vi "ADC_spb.vi"(1 "18_1":i8=18, 2 "18_1":i8=18, 3 "8":i8=8, 4 "7":i8=7, 5 "Write Data":bool[](array[boolean])=[FALSE, FALSE, FALSE, FALSE, FALSE, FALSE, FALSE, FALSE, FALSE], 6 "Enum":T1(ring)=enum."GREEN OFF", 7 "Read(T)/Write(F)":bool, 8 "Command array":bool[](array[boolean])=[FALSE, FALSE, FALSE, FALSE, FALSE, FALSE, FALSE, FALSE, FALSE, FALSE, FALSE, FALSE, FALSE, FALSE, FALSE, FALSE, FALSE]) -> (0 "READ":bool[](array[boolean]))   [LabVIEW 2018]
uses:
  <vilib>/Platform/TimedLoop/XDataNode/timing_clust.ctl
  <vilib>/Platform/TimedLoop/XDataNode/nitl_modes.ctl
  <vilib>/Platform/TimedLoop/XDataNode/wakeup.ctl
  <vilib>/rvi/Emulation/niFpgaSctlEmulationGetInTimedLoop.vi
  <vilib>/rvi/Emulation/niFpgaEmulationReportErrorSimple.vi
  <vilib>/rvi/Emulation/niFpgaGetClockAttributes.vi
  <vilib>/rvi/Emulation/niFpgaCriticalErrorInLSC.vi
  <vilib>/rvi/eio/common/nirviEmuTemplateMethod_errors.vi
  <vilib>/Platform/TimedLoop/XDataNode/XDataNode.xnode
  <vilib>/eio/EIONode/EIONode.xnode
  <vilib>/Platform/TimedLoop/XDataNode/XDNodeRunTimeDep.lvlib
panel:
  in  "17":i8=17
  # "8"
  # "0"
  # "8"
  # "0"
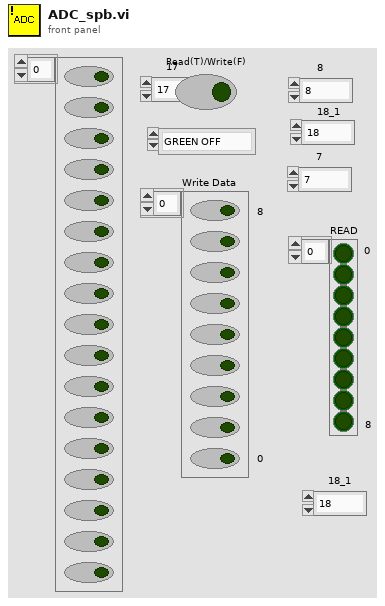
[diagram p1: front panel]
types:
  T1 = enum16{"Configuration", "MUX", "RED PGA", "GREEN PGA", "BLUE PGA", "RED OFF", "GREEN OFF", "BLUE OFF"}
  T2 = typedef "XDNodeRunTimeDep.lvlib/timing_clust.ctl" = cluster{"Expected End [f-1]":u64, "Actual End [f-1]":u64, "Finished Late? [f-1]":bool, "Expected End [i-1]":u64, "Actual End [i-1]":u64, "Finished Late? [i-1]":bool, "Expected Start [i]":u64, "Actual Start [i]":u64, "Expected Start [f]":u64, "Actual Start [f]":u64, "Source Name":string, "Structure Name":string, "Period":i64, "Deadline":i64, "Offset":i64, "Start":i64, "Priority":i32, "Timeout":i32, "Mode":T3, "Wakeup Reason":T4, "Error":errorcluster, "Source Type":string, "Secondary Source Type":string, "Global End Time":u64, "Global Start Time":u64, "Frame Duration":u64, "Iteration Duration":u64, "Assigned CPU":i32, "I/O Scan Engine Mode":u32}
  T3 = typedef "XDNodeRunTimeDep.lvlib/nitl_modes.ctl" = enum32{"No Change", "Process missed periods, maintain original phase", "Discard missed periods, maintain original phase", "Process missed periods, ignore original phase", "Discard missed periods, ignore original phase"}
  T4 = typedef "XDNodeRunTimeDep.lvlib/wakeup.ctl" = enum32{"Normal", "Aborted", "Asynchronous wakeup", "Timing source error", "Timed loop error", "Timeout"}
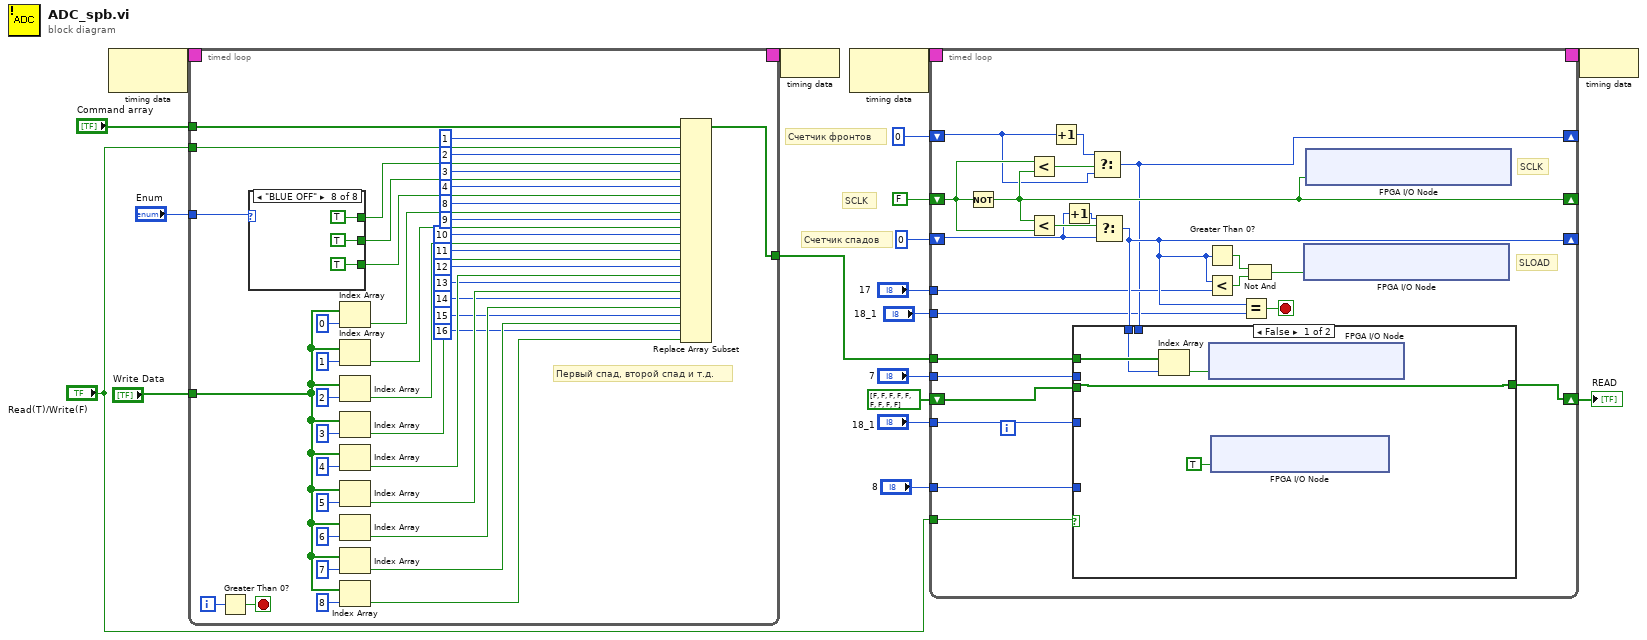
[diagram p0: block diagram]
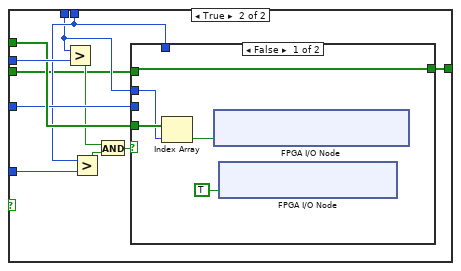
[diagram p2: hidden frame]
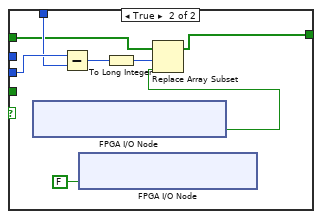
[diagram p3: hidden frame]
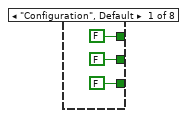
[diagram p4: hidden frame]
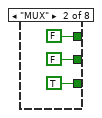
[diagram p5: hidden frame]
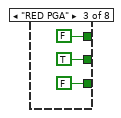
[diagram p6: hidden frame]
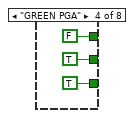
[diagram p7: hidden frame]
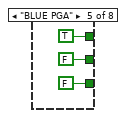
[diagram p8: hidden frame]
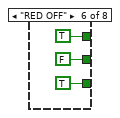
[diagram p9: hidden frame]
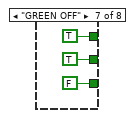
[diagram p10: hidden frame]
diagram:
  # "Счетчик фронтов"
  # "Счетчик спадов"
  # "SCLK"
  n1 = node-c288() -> (w19:T2)  [unwired: 1 in]
  n2 = timed-loop {
    timing: w19 -> [_]
    timing-out: [_] -> w18
    tunnel: "Enum" -> [w51]
    tunnel: "Command array" -> [w46]
    tunnel: [w50] -> w10
    tunnel: "Read(T)/Write(F)" -> [w44]
    tunnel: "Write Data" -> [w49]
    i -> [w47]
    stop <- w48 stop-if-true
    # "Первый спад, второй спад и т.д."
    n3 = Greater Than 0?(x=w47) -> (x > 0?=w48:bool)
    n4 = case shown="\"BLUE OFF\"" w51 {
      tunnel: [FALSE FALSE FALSE FALSE TRUE TRUE TRUE TRUE] -> w42
      tunnel: [FALSE FALSE TRUE TRUE FALSE FALSE TRUE TRUE] -> w41
      tunnel: [FALSE TRUE FALSE TRUE FALSE TRUE FALSE TRUE] -> w40
      frame "Configuration", Default {
      }
      frame "MUX" {
      }
      frame "RED PGA" {
      }
      frame "GREEN PGA" {
      }
      frame "BLUE PGA" {
      }
      frame "RED OFF" {
      }
      frame "GREEN OFF" {
      }
      frame "BLUE OFF" {
      }
    }
    n5 = Index Array(array=w49, index=0) -> (element=w37:bool)
    n6 = Index Array(array=w49, index=1) -> (element=w36:bool)
    n7 = Index Array(array=w49, index=2) -> (element=w35:bool)
    n8 = Index Array(array=w49, index=3) -> (element=w34:bool)
    n9 = Index Array(array=w49, index=4) -> (element=w33:bool)
    n10 = Index Array(array=w49, index=5) -> (element=w32:bool)
    n11 = Index Array(array=w49, index=6) -> (element=w31:bool)
    n12 = Index Array(array=w49, index=7) -> (element=w30:bool)
    n13 = Index Array(array=w49, index=8) -> (element=w29:bool)
    n14 = Replace Array Subset(array=w46, new element #1=w44, index #1=1 ("index"), new element #2=w42, index #2=2 ("index"), new element #3=w41, index #3=3 ("index"), new element #4=w40, index #4=4 ("index"), new element #5=w37, index #5=8 ("index"), new element #6=w36, index #6=9 ("index"), new element #7=w35, index #7=10 ("index"), new element #8=w34, index #8=11 ("index"), new element #9=w33, index #9=12 ("index"), new element #10=w32, index #10=13 ("index"), new element #11=w31, index #11=14 ("index"), new element #12=w30, index #12=15 ("index"), new element #13=w29, index #13=16 ("index")) -> (w50:bool[])
  }
  n15 = node-c288(w18) -> ()
  n16 = node-c288() -> (w17:T2)  [unwired: 1 in]
  n17 = timed-loop {
    timing: w17 -> [_]
    timing-out: [_] -> w16
    shift-right: [w96] -> _
    shift-left: FALSE -> [w97]
    shift-right: [w100] -> _
    shift-left: i8 0 -> [w107]
    tunnel: w10 -> [w103]
    tunnel: "17" -> [w99]
    tunnel: "7" -> [w102]
    tunnel: "Read(T)/Write(F)" -> [w101]
    shift-right: [w92] -> _
    shift-left: i8 0 -> [w93]
    tunnel: "18_1" -> [w91]
    tunnel: "8" -> [w90]
    shift-right: [w88] -> w3
    shift-left: bool[] [FALSE, FALSE, FALSE, FALSE, FALSE, FALSE, FALSE, FALSE, FALSE] -> [w89]
    tunnel: "18_1" -> [w87]
    stop <- w98 stop-if-true
    # "SLOAD"
    # "SCLK"
    n18 = Not(x=w97) -> (.not. x?=w96:bool)
    n19 = Less?(x=w97, y=w96) -> (x < y?=w95:bool)
    n20 = Less?(x=w96, y=w97) -> (x < y?=w109:bool)
    n21 = Increment(x=w93) -> (x+1=w94:i8)
    n22 = Increment(x=w107) -> (x+1=w108:i8)
    n23 = Select(t=w94, s=w95, f=w93) -> (s? t:f=w92:i8)
    n24 = Select(t=w108, s=w109, f=w107) -> (s? t:f=w100:i8)
    n25 = case shown="False" w101 {
      tunnel: w103 -> [w114 w124]
      tunnel: w100 -> [w113 w117]
      tunnel: w102 -> [_ w125]
      tunnel: w92 -> [_ w121]
      tunnel: w91 -> [_ w123]
      tunnel: w90 -> [_ w120]
      tunnel: w89 -> [w110 w116]
      tunnel: [w110 w115] -> w88
      frame False {
        n26 = Index Array(array=w114, index=w113) -> (element=w112:bool)
        n27 = xnode "FPGA I/O Node"("IO Module\\DDCB_PFI1_Write"=w112) -> ()  [unwired: 1 in, 1 out]
        n28 = xnode "FPGA I/O Node"("IO Module\\DDCB_PFI_WE"=TRUE ("IO Module\\DDCA_PFI_WE")) -> ()  [unwired: 1 in, 1 out]
      }
      frame True {
        n29 = Greater?(x=w117, y=w125) -> (0:w122:bool)
        n30 = Greater?(x=w121, y=w120) -> (0:w119:bool)
        n31 = And(x=w122, y=w119) -> (x .and. y?=w118:bool)
        n32 = case shown="False" w118 {
          tunnel: w124 -> [w130 _]
          tunnel: w121 -> [_ w135]
          tunnel: w123 -> [_ w136]
          tunnel: w117 -> [w127 _]
          tunnel: w116 -> [w126 w132]
          tunnel: [w126 w131] -> w115
          frame False {
            n33 = Index Array(array=w130, index=w127) -> (element=w128:bool)
            n34 = xnode "FPGA I/O Node"("IO Module\\DDCB_PFI1_Write"=w128) -> ()  [unwired: 1 in, 1 out]
            n35 = xnode "FPGA I/O Node"("IO Module\\DDCB_PFI_WE"=TRUE ("IO Module\\DDCA_PFI_WE")) -> ()  [unwired: 1 in, 1 out]
          }
          frame True {
            n36 = xnode "FPGA I/O Node"() -> ("IO Module\\DDCB_PFI1_Read"=w137:bool)  [unwired: 1 in, 1 out]
            n37 = Subtract(x=w136, y=w135) -> (x-y=w133:i8)
            n38 = xnode "FPGA I/O Node"("IO Module\\DDCB_PFI_WE"=FALSE ("IO Module\\DDCA_PFI_WE")) -> ()  [unwired: 1 in, 1 out]
            n39 = To Long Integer(number=w133) -> (32bit integer=w134:i32)
            n40 = Replace Array Subset(array=w132, new element=w137, index=w134) -> (w131:bool[])
          }
        }
      }
    }
    n41 = Greater Than 0?(x=w100) -> (x > 0?=w106:bool)
    n42 = Less?(x=w100, y=w99) -> (x < y?=w105:bool)
    n43 = Equal?(x=w100, y=w87) -> (x = y?=w98:bool)
    n44 = Not And(1:w105, 2:w106) -> (0:w104:bool)
    n45 = xnode "FPGA I/O Node"("IO Module\\DDCB_DIO15_Write"=w104) -> ()  [unwired: 1 in, 1 out]
    n46 = xnode "FPGA I/O Node"("IO Module\\DDCB_DIO14_Write"=w96) -> ()  [unwired: 1 in, 1 out]
  }
  "READ" <- w3
  n47 = node-c288(w16) -> ()
